vi "add_to_file.vi"(8 "error in (no error)":errorcluster, 9 "Add return?":bool=TRUE, 10 "String":string, 11 "Path to log":path) -> (0 "error out":errorcluster)   [LabVIEW 2017, in "DataLogging.lvclass"]
doc: "adds the string add the end of the file given in path. if the file doesn't exist, the subviw creates it."
uses:
  DataLogging.lvclass
  <vilib>/Utility/error.llb/DialogType.ctl
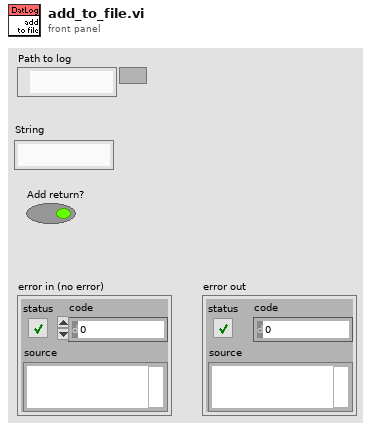
[diagram p1: front panel]
types:
  T1 = typedef "DialogType.ctl" = u16
  T2 = enum16{"open", "replace", "create", "open or create", "replace or create", "replace or create with confirmation"}
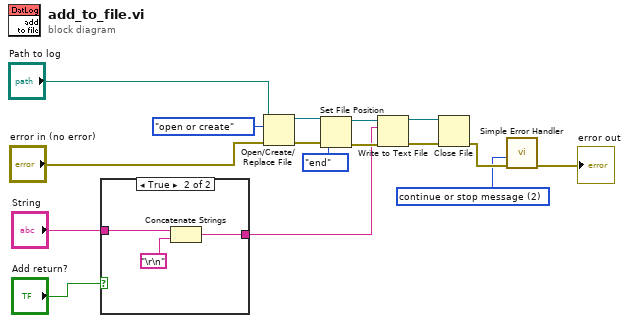
[diagram p0: block diagram]
diagram:
  w1 = T1 2 items=["no dialog", "OK message", "continue or stop message", "OK message + warnings", "continue/stop + warnings"] ("type of dialog (OK msg:1)")
  n1 = case shown="True" "Add return?" {
    tunnel: "String" -> [w17 w20]
    tunnel: [w17 w18] -> w3
    frame False {
    }
    frame True {
      n2 = Concatenate Strings(w20, "\r\n") -> (w18:string)
    }
  }
  n3 = Open/Create/Replace File(file path (use dialog)="Path to log", error in="error in (no error)", operation (0:open)=T2."open or create") -> (refnum out=w10:refnum<file>, error out=w11:errorcluster)  [unwired: 3 in, 1 out]
  n4 = Set File Position(refnum=w10, from (0:start)=enum16{"start", "end", "current"}."end", error in=w11) -> (refnum out=w13:refnum<file>, error out=w14:errorcluster)  [unwired: 1 in]
  n5 = Write to Text File(file (use dialog)=w13, text=w3, error in=w14) -> (refnum out=w16:refnum<file>, error out=w15:errorcluster)  [unwired: 1 in, 1 out]
  n6 = Close File(refnum=w16, error in=w15) -> (error out=w6:errorcluster)  [unwired: 1 out]
  n7 = call <vilib>:"Simple Error Handler.vi"("type of dialog (OK msg:1)"=w1, "error in (no error)"=w6) -> ("error out"=→"error out":errorcluster)  [unwired: 3 in, 4 out]
